vi "GEOM_Read_FPAReadModes.vi"(8 "error in (no error)":errorcluster, 11 "file path":path) -> (0 "error out":errorcluster, 2 "FPAReadModes":T1(array[cluster]), 3 "file path out":path)   [LabVIEW 2016]
uses:
  <vilib>/Utility/config.llb/Read Key (String).vi
  <vilib>/Utility/config.llb/NI_LVConfig.lvlib
panel:
  in  "section":string="FPAREADMODES"
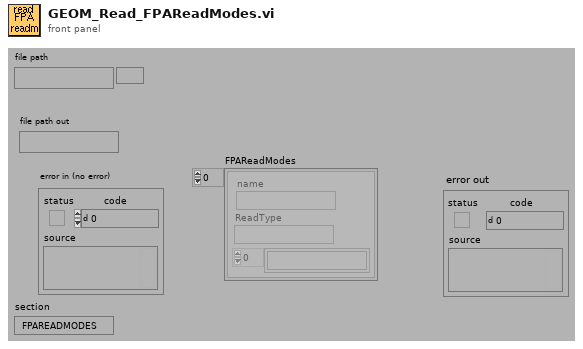
[diagram p1: front panel]
types:
  T1 = cluster{"name":string, "ReadType":string, string[]}[]
  T2 = typedef "NI_LVConfig.lvlib/Config Data RefNum.ctl" = refnum<k1>
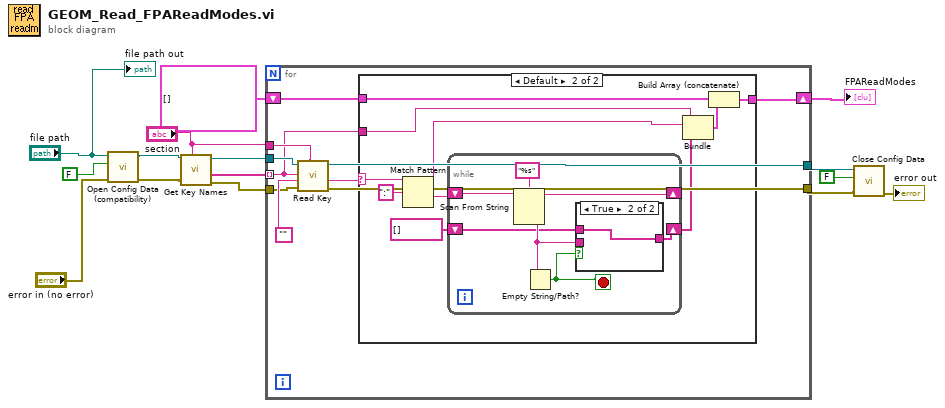
[diagram p0: block diagram]
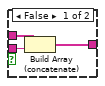
[diagram p3: hidden frame]
diagram:
  n1 = call <vilib>:"Open Config Data (compatibility).vi"("error in (no error)"="error in (no error)", "create file if necessary (T)"=FALSE ("create file if necessary? (T)"), "configuration file path"="file path") -> ("error out"=w13:errorcluster, "refnum"=w14:T2)  [unwired: 6 in, 1 out]
  n2 = call <vilib>:"Get Key Names.vi"("section"="section", "error in (no error)"=w13, "refnum"=w14) -> ("error out"=w9:errorcluster, "key names"=w12:string[], "refnum out"=w11:T2)  [unwired: 6 out]
  n3 = for {
    tunnel: w12 -> [w22] mode=indexing
    tunnel: "section" -> [w25]
    tunnel: w11 -> [w24]
    tunnel: [w21] -> w10
    tunnel: w9 -> [w20]
    tunnel: [w19] -> w8
    shift-right: [w17] -> w2
    shift-left: cluster{"String":string, string, string[]}[] [] -> [w16]
    n4 = call-poly <vilib>:"Read Key.vi"("section"=w25, "error in (no error)"=w20, "default value"="", "key"=w22, "refnum"=w24) -> ("error out"=w19:errorcluster, "value"=w18:string, "refnum out"=w21:T2)  [unwired: 1 in, 3 out]
    n5 = case shown="Default" w18 {
      selector: w18 -> [_ w36]
      tunnel: w22 -> [_ w30]
      tunnel: [w26 w28] -> w17
      tunnel: w16 -> [w26 w27]
      frame "", " " {
      }
      frame Default {
        n6 = Match Pattern(string=w36, regular expression=":") -> (before substring=w32:string, after substring=w34:string)  [unwired: 3 out]
        n7 = while {
          shift-right: [w42] -> _
          shift-left: w34 -> [w37]
          shift-right: [w38] -> w31
          shift-left: string[] [] -> [w39]
          stop <- w41 stop-if-true
          n8 = Scan From String(format string="%s", input string=w37) -> (remaining string=w42:string, output 1=w40:string)  [unwired: 2 in, 3 out]
          n9 = Empty String/Path?(string/path=w40) -> (empty?=w41:bool)
          n10 = case shown="True" w41 {
            tunnel: w40 -> [w46 _]
            tunnel: w39 -> [w45 w47]
            tunnel: [w44 w47] -> w38
            frame False {
              n11 = Build Array (concatenate)(w45, w46) -> (w44:string[])
            }
            frame True {
            }
          }
        }
        n12 = Bundle("String"=w30, w32, w31) -> (w29:cluster{"String":string, string, string[]})  [unwired: 1 out]
        n13 = Build Array (concatenate)(w27, w29) -> (w28:cluster{"String":string, string, string[]}[])
      }
    }
  }
  "FPAReadModes" <- w2
  n14 = call <vilib>:"Close Config Data.vi"("error in (no error)"=w8, "write file if changed (T)"=FALSE ("write configuration file? (F)"), "refnum"=w10) -> ("error out"=→"error out":errorcluster)  [unwired: 8 out]
  "file path out" <- "file path"
